vi "Unflatten-TouchFingerEventData.vi"(8 "error in (no error)":errorcluster, 11 "Event Binary Data":string) -> (0 "error out":errorcluster, 3 "Event Data":T1)   [LabVIEW 2026, in "SDL3.lvlib" / "Events.lvlib"]
uses:
  TouchFingerEventData--cluster.ctl
  Joystick/JoystickID--integer.ctl
  Touch/FingerID--integer.ctl
  Video/WindowID--integer.ctl
  Events.lvlib
  Joystick/Joystick.lvlib
  Touch/Touch.lvlib
  Video/Video.lvlib
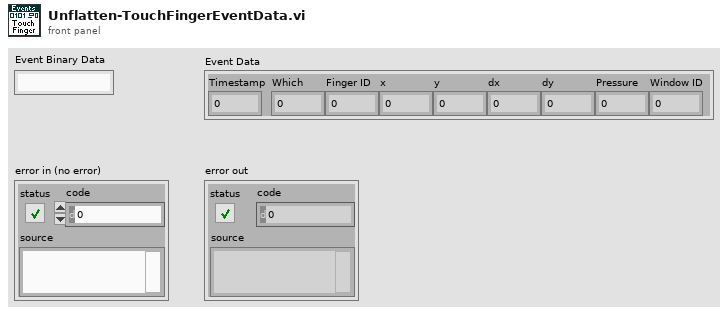
[diagram p1: front panel]
types:
  T1 = typedef "SDL3.lvlib/Events.lvlib/TouchFingerEventData--cluster.ctl" = cluster{"Timestamp":u64, "Which":T2, "Finger ID":T3, "x":sgl, "y":sgl, "dx":sgl, "dy":sgl, "Pressure":sgl, "Window ID":T4}
  T2 = typedef "SDL3.lvlib/Joystick.lvlib/JoystickID--integer.ctl" = u32
  T3 = typedef "SDL3.lvlib/Touch.lvlib/FingerID--integer.ctl" = u64
  T4 = typedef "SDL3.lvlib/Video.lvlib/WindowID--integer.ctl" = u32
  T5 = enum16{"big-endian, network order", "native, host order", "little-endian"}
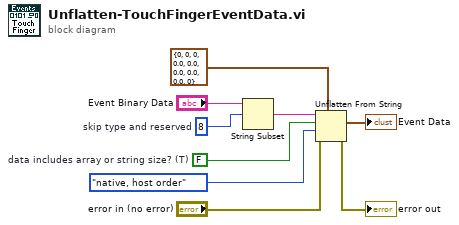
[diagram p0: block diagram]
diagram:
  w3 = 8  # skip type and reserved
  w6 = FALSE  # data includes array or string size? (T)
  n1 = String Subset(string="Event Binary Data", offset (0)=w3) -> (substring=w4:string)  [unwired: 1 in]
  n2 = Unflatten From String(type=T1 {"Timestamp"=0, "Which"=0, "Finger ID"=0, "x"=0.0, "y"=0.0, "dx"=0.0, "dy"=0.0, "Pressure"=0.0, "Window ID"=0} ("TouchFingerEvent"), binary string=w4, data includes array or string size? (T)=w6, byte order (0:big-endian, network order)=T5."native, host order", error in (no error)="error in (no error)") -> (value=→"Event Data":T1, error out=→"error out":errorcluster)  [unwired: 1 out]
